vi "Lab_2_START_Arrays_String_ShiftRegisters (3) (1).vi"() -> ()   [LabVIEW 2025]
panel:
  out "BPM":cluster{"Time":timestamp[], "Bpm":i32[]}(graph)
  out "HEART RATE ZONES 2":T1(graph)
  out "HEART RATE ZONES":string[][](array[string])
  in  "Age":i32
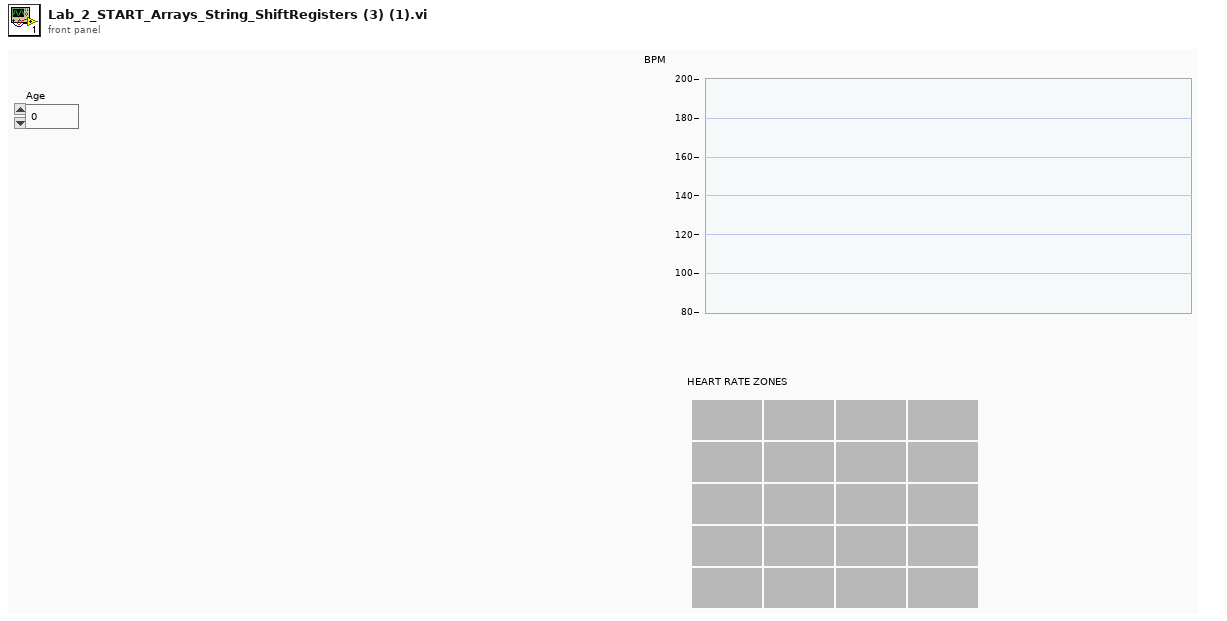
[diagram p1: front panel]
types:
  T1 = cluster{" Total time in Zone (%) ":dbl[], "Heart Rate Zone":i32[]}
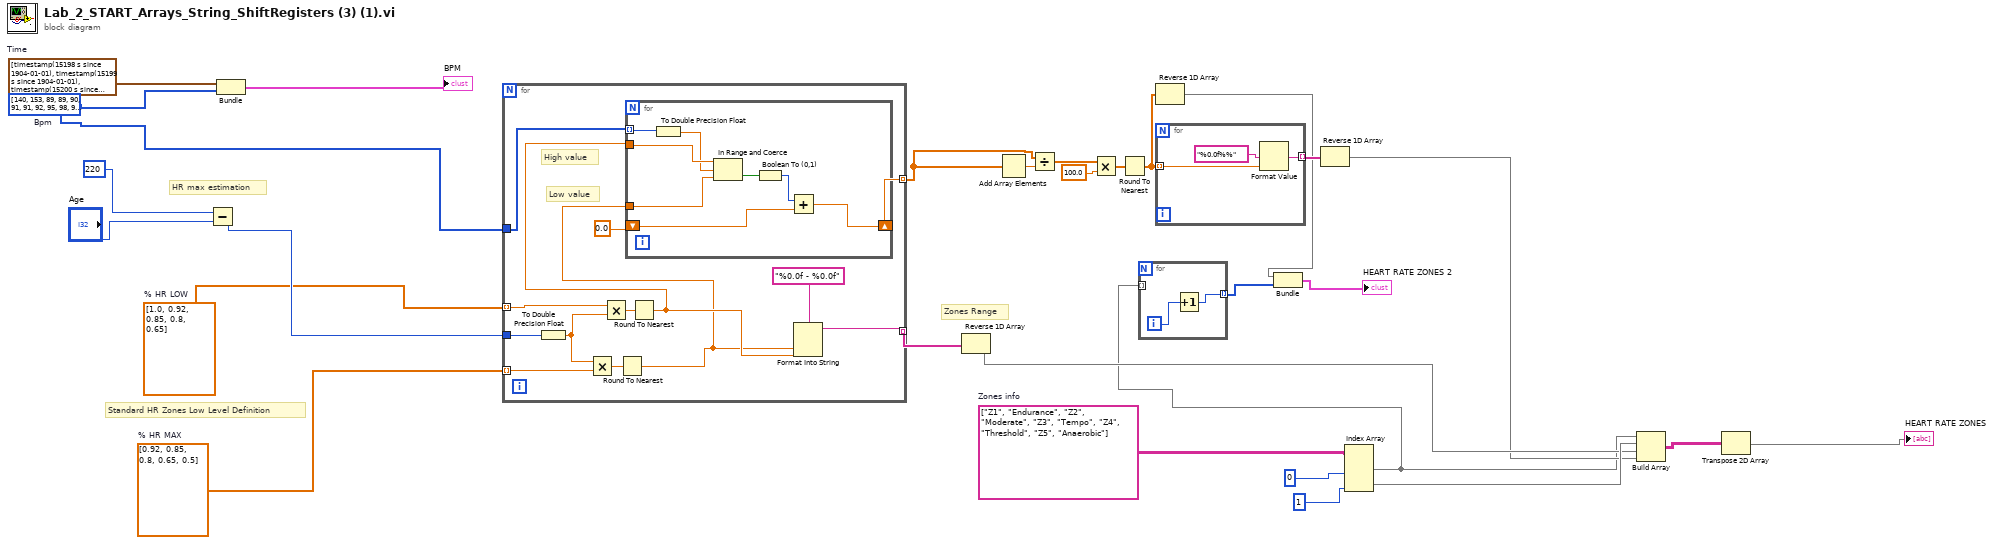
[diagram p0: block diagram]
diagram:
  w24 = dbl[] [1.0, 0.92, 0.85, 0.8, 0.65]  # % HR LOW
  w4 = i32[] [140, 153, 89, 89, 90, 91, 91, 92, 95, 98, 99, 103, 105, 112, 112, 113, 116, 117, 120, 123, 124, 127, 128, 129, 129, 129, 132, 132, 132, 133, 132, 135, 136, 137, 137, 136, 137, 138, 142, 142, 143, 146, 145, 145, 146, 146, 145, 146, 149, 146, 148, 145, 145, 146, 147, 147, 146, 145, 145, 146, 146, 146, 147, 148, 146, 146, 144, 143, 143, 143, 141, 141, 140, 142, 143, 144, 143, 143, 143, 143, 146, 146, 146, 146, 149, 149, 150, 152, 152, 152, 152, 153, 151, 150, 151, 151, 150, 150, 151, 151, 150, 151, 151, 151, 150, 151, 150, 148, 148, 148, 147, 157, 147, 147, 147, 148, 150, 151, 152, 152, 154, 154, 155, 155, 154, 154, 153, 153, 153, 153, 152, 149, 149, 149, 148, 147, 147, 147, 146, 146, 146, 147, 144, 143, 142, 141, 140, 141, 142, 142, 142, 141, 141, 142, 141, 140, 140, 140, 140, 140, 140, 140, 140, 139, 140, 139, 139, 139, 138, 140, 142, 141, 141, 142, 143, 143, 143, 139, 139, 140, 140, 142, 144, 145, 147, 148, 149, 150, 152, 152, 152, 153, 153, 154, 154, 155, 155, 156, 157, 156, 156, 155, 155, 151, 155, 154, 154, 153, 152, 152, 152, 152, 152, 152, 151, 151, 150, 150, 151, 150, 151, 150, 151, 151, 152, 152, 151, 152, 151, 150, 152, 151, 151, 150, 150, 149, 148, 148, 148, 148, 149, 150, 151, 151, 149, 149, 148, 148, 148, 150, 152, 152, 153, 151, 151, 151, 152, 153, 153, 152, 151, 151, 152, 151, 151, 151, 152, 152, 153, 167, 173, 153, 155, 157, 158, 159, 160, 160, 159, 159, 160, 161, 161, 162, 161, 162, 163, 164, 165, 165, 164, 165, 165, 166, 167, 167, 167, 167, 168, 167, 167, 167, 168, 168, 168, 168, 169, 169, 169, 170, 169, 172, 173, 170, 171, 171, 172, 172, 171, 171, 171, 171, 171, 171, 169, 166, 172, 173, 172, 173, 172, 172, 172, 172, 172, 172, 173, 172, 173, 172, 172, 172, 172, 172, 172, 171, 172, 172, 172, 129, 173, 172, 172, 173, 169, 166, 166, 166, 164, 163, 162, 161, 161, 157, 156, 154, 150, 149, 146, 143, 140, 137, 138, 137, 135, 135, 134, 135, 132, 131, 129, 128, 126, 126, 125, 126, 123, 123, 125, 124, 120, 118, 118, 116, 116, 116, 116, 116, 116, 115, 116, 114, 115, 117, 116, 116, 115, 114, 116, 116, 113, 112, 112, 112, 113, 116, 118, 121, 164, 176, 121, 125, 129, 133, 136, 139, 141, 144, 146, 149, 150, 153, 153, 156, 156, 157, 159, 161, 161, 163, 163, 164, 164, 164, 164, 166, 165, 167, 168, 168, 168, 167, 168, 168, 169, 169, 169, 170, 171, 171, 172, 171, 174, 172, 173, 171, 174, 173, 172, 172, 172, 172, 173, 173, 172, 173, 174, 173, 174, 174, 174, 174, 175, 175, 175, 175, 175, 136, 175, 175, 175, 174, 173, 173, 170, 169, 165, 164, 164, 163, 163, 160, 157, 154, 151, 150, 147, 144, 144, 141, 138, 137, 134, 133, 134, 131, 129, 128, 127, 126, 126, 124, 123, 122, 122, 124, 123, 122, 121, 120, 119, 119, 119, 119, 123, 125, 124, 124, 122, 124, 127, 130, 133, 134, 162, 172, 134, 137, 138, 142, 145, 145, 147, 150, 150, 151, 153, 155, 157, 160, 160, 162, 163, 164, 164, 165, 167, 167, 168, 168, 169, 169, 170, 170, 170, 170, 170, 170, 170, 170, 171, 171, 171, 172, 171, 156, 172, 171, 170, 168, 168, 168, 166, 166, 165, 164, 163, 164, 163, 163, 163, 162, 162, 160, 159, 159, 158, 156, 156, 155, 152, 152, 152, 151, 149, 149, 149, 149, 148, 147, 148, 148, 148, 149, 148, 148, 148, 149, 149, 151, 151, 161, 166, 151, 153, 153, 156, 158, 161, 162, 161, 163, 165, 166, 166, 153, 166, 166, 165, 162, 162, 161, 160, 157, 155, 152, 151, 151, 152, 152, 151, 151, 149, 148, 148, 148, 155, 159, 148, 149, 152, 153, 155, 158, 158, 159, 159, 156, 159, 159, 159, 158, 158, 158, 158, 157, 157, 155, 155, 155, 154, 154, 152, 153, 160, 165, 153, 153, 153, 156, 156, 158, 160, 162, 164, 165, 165, 165, 155, 165, 165, 164, 161, 160, 159, 159, 156, 156, 155, 155, 154, 154, 154, 153, 153, 153, 151, 150, 151, 151, 161, 167, 151, 154, 156, 159, 160, 163, 163, 166, 167, 166, 157, 166, 166, 165, 162, 162, 162, 162, 161, 160, 159, 159, 157, 156, 156, 153, 154, 153, 151, 150, 151, 153, 160, 164, 153, 156, 158, 160, 161, 162, 162, 163, 163, 165, 151, 165, 165, 165, 162, 162, 161, 160, 159, 158, 156, 155, 152, 151, 151, 150, 150, 146, 144, 145, 145, 145, 146, 147, 148, 158, 166, 148, 152, 153, 156, 158, 160, 163, 164, 166, 166, 151, 167, 166, 164, 161, 158, 157, 156, 155, 154, 154, 151, 150, 149, 146, 145, 143, 142, 139, 139, 138, 138, 135, 137, 155, 160, 137, 137, 139, 139, 140, 141, 142, 143, 145, 146, 148, 150, 152, 153, 153, 155, 156, 156, 158, 158, 159, 158, 158, 159, 159, 159, 159, 159, 159, 159, 159, 159, 159, 159, 159, 159, 159, 158, 157, 157, 158, 158, 157, 156, 156, 155, 157, 156, 156, 157, 157, 156, 156, 156, 156, 157, 156, 155, 155, 155, 156, 156, 159, 159, 158, 158, 157, 157, 158, 158, 158, 158, 159, 158, 158, 158, 157, 157, 157, 156, 156, 156, 154, 154, 154, 154, 156, 155, 157, 157, 157, 157, 158, 158, 158, 159]  # Bpm
  w28 = timestamp[] [timestamp(15198 s since 1904-01-01), timestamp(15199 s since 1904-01-01), timestamp(15200 s since 1904-01-01), timestamp(15202 s since 1904-01-01), timestamp(15203 s since 1904-01-01), timestamp(15207 s since 1904-01-01), timestamp(15209 s since 1904-01-01), timestamp(15211 s since 1904-01-01), timestamp(15213 s since 1904-01-01), timestamp(15215 s since 1904-01-01), timestamp(15218 s since 1904-01-01), timestamp(15220 s since 1904-01-01), timestamp(15221 s since 1904-01-01), timestamp(15223 s since 1904-01-01), timestamp(15226 s since 1904-01-01), timestamp(15227 s since 1904-01-01), timestamp(15229 s since 1904-01-01), timestamp(15231 s since 1904-01-01), timestamp(15235 s since 1904-01-01), timestamp(15241 s since 1904-01-01), timestamp(15244 s since 1904-01-01), timestamp(15245 s since 1904-01-01), timestamp(15248 s since 1904-01-01), timestamp(15250 s since 1904-01-01), timestamp(15256 s since 1904-01-01), timestamp(15257 s since 1904-01-01), timestamp(15258 s since 1904-01-01), timestamp(15263 s since 1904-01-01), timestamp(15265 s since 1904-01-01), timestamp(15267 s since 1904-01-01), timestamp(15269 s since 1904-01-01), timestamp(15274 s since 1904-01-01), timestamp(15275 s since 1904-01-01), timestamp(15277 s since 1904-01-01), timestamp(15279 s since 1904-01-01), timestamp(15285 s since 1904-01-01), timestamp(15291 s since 1904-01-01), timestamp(15294 s since 1904-01-01), timestamp(15299 s since 1904-01-01), timestamp(15301 s since 1904-01-01), timestamp(15302 s since 1904-01-01), timestamp(15308 s since 1904-01-01), timestamp(15313 s since 1904-01-01), timestamp(15319 s since 1904-01-01), timestamp(15320 s since 1904-01-01), timestamp(15324 s since 1904-01-01), timestamp(15329 s since 1904-01-01), timestamp(15335 s since 1904-01-01), timestamp(15337 s since 1904-01-01), timestamp(15341 s since 1904-01-01), timestamp(15343 s since 1904-01-01), timestamp(15348 s since 1904-01-01), timestamp(15354 s since 1904-01-01), timestamp(15355 s since 1904-01-01), timestamp(15356 s since 1904-01-01), timestamp(15362 s since 1904-01-01), timestamp(15364 s since 1904-01-01), timestamp(15370 s since 1904-01-01), timestamp(15373 s since 1904-01-01), timestamp(15376 s since 1904-01-01), timestamp(15379 s since 1904-01-01), timestamp(15381 s since 1904-01-01), timestamp(15387 s since 1904-01-01), timestamp(15392 s since 1904-01-01), timestamp(15398 s since 1904-01-01), timestamp(15402 s since 1904-01-01), timestamp(15405 s since 1904-01-01), timestamp(15411 s since 1904-01-01), timestamp(15412 s since 1904-01-01), timestamp(15418 s since 1904-01-01), timestamp(15424 s since 1904-01-01), timestamp(15426 s since 1904-01-01), timestamp(15428 s since 1904-01-01), timestamp(15433 s since 1904-01-01), timestamp(15436 s since 1904-01-01), timestamp(15440 s since 1904-01-01), timestamp(15446 s since 1904-01-01), timestamp(15447 s since 1904-01-01), timestamp(15450 s since 1904-01-01), timestamp(15451 s since 1904-01-01), timestamp(15452 s since 1904-01-01), timestamp(15453 s since 1904-01-01), timestamp(15456 s since 1904-01-01), timestamp(15458 s since 1904-01-01), timestamp(15459 s since 1904-01-01), timestamp(15465 s since 1904-01-01), timestamp(15466 s since 1904-01-01), timestamp(15468 s since 1904-01-01), timestamp(15471 s since 1904-01-01), timestamp(15472 s since 1904-01-01), timestamp(15477 s since 1904-01-01), timestamp(15483 s since 1904-01-01), timestamp(15484 s since 1904-01-01), timestamp(15486 s since 1904-01-01), timestamp(15491 s since 1904-01-01), timestamp(15494 s since 1904-01-01), timestamp(15498 s since 1904-01-01), timestamp(15504 s since 1904-01-01), timestamp(15509 s since 1904-01-01), timestamp(15515 s since 1904-01-01), timestamp(15516 s since 1904-01-01), timestamp(15521 s since 1904-01-01), timestamp(15522 s since 1904-01-01), timestamp(15525 s since 1904-01-01), timestamp(15531 s since 1904-01-01), timestamp(15537 s since 1904-01-01), timestamp(15538 s since 1904-01-01), timestamp(15540 s since 1904-01-01), timestamp(15546 s since 1904-01-01), timestamp(15547 s since 1904-01-01), timestamp(15548 s since 1904-01-01), timestamp(15552 s since 1904-01-01), timestamp(15556 s since 1904-01-01), timestamp(15559 s since 1904-01-01), timestamp(15562 s since 1904-01-01), timestamp(15568 s since 1904-01-01), timestamp(15573 s since 1904-01-01), timestamp(15574 s since 1904-01-01), timestamp(15580 s since 1904-01-01), timestamp(15581 s since 1904-01-01), timestamp(15583 s since 1904-01-01), timestamp(15586 s since 1904-01-01), timestamp(15592 s since 1904-01-01), timestamp(15596 s since 1904-01-01), timestamp(15597 s since 1904-01-01), timestamp(15603 s since 1904-01-01), timestamp(15608 s since 1904-01-01), timestamp(15612 s since 1904-01-01), timestamp(15613 s since 1904-01-01), timestamp(15619 s since 1904-01-01), timestamp(15621 s since 1904-01-01), timestamp(15623 s since 1904-01-01), timestamp(15627 s since 1904-01-01), timestamp(15629 s since 1904-01-01), timestamp(15633 s since 1904-01-01), timestamp(15634 s since 1904-01-01), timestamp(15639 s since 1904-01-01), timestamp(15641 s since 1904-01-01), timestamp(15646 s since 1904-01-01), timestamp(15650 s since 1904-01-01), timestamp(15653 s since 1904-01-01), timestamp(15656 s since 1904-01-01), timestamp(15660 s since 1904-01-01), timestamp(15664 s since 1904-01-01), timestamp(15668 s since 1904-01-01), timestamp(15669 s since 1904-01-01), timestamp(15671 s since 1904-01-01), timestamp(15675 s since 1904-01-01), timestamp(15676 s since 1904-01-01), timestamp(15678 s since 1904-01-01), timestamp(15683 s since 1904-01-01), timestamp(15689 s since 1904-01-01), timestamp(15690 s since 1904-01-01), timestamp(15694 s since 1904-01-01), timestamp(15695 s since 1904-01-01), timestamp(15699 s since 1904-01-01), timestamp(15700 s since 1904-01-01), timestamp(15701 s since 1904-01-01), timestamp(15704 s since 1904-01-01), timestamp(15707 s since 1904-01-01), timestamp(15711 s since 1904-01-01), timestamp(15713 s since 1904-01-01), timestamp(15714 s since 1904-01-01), timestamp(15718 s since 1904-01-01), timestamp(15724 s since 1904-01-01), timestamp(15730 s since 1904-01-01), timestamp(15734 s since 1904-01-01), timestamp(15736 s since 1904-01-01), timestamp(15742 s since 1904-01-01), timestamp(15746 s since 1904-01-01), timestamp(15752 s since 1904-01-01), timestamp(15754 s since 1904-01-01), timestamp(15759 s since 1904-01-01), timestamp(15764 s since 1904-01-01), timestamp(15769 s since 1904-01-01), timestamp(15770 s since 1904-01-01), timestamp(15775 s since 1904-01-01), timestamp(15779 s since 1904-01-01), timestamp(15781 s since 1904-01-01), timestamp(15784 s since 1904-01-01), timestamp(15789 s since 1904-01-01), timestamp(15791 s since 1904-01-01), timestamp(15794 s since 1904-01-01), timestamp(15800 s since 1904-01-01), timestamp(15805 s since 1904-01-01), timestamp(15806 s since 1904-01-01), timestamp(15809 s since 1904-01-01), timestamp(15813 s since 1904-01-01), timestamp(15814 s since 1904-01-01), timestamp(15820 s since 1904-01-01), timestamp(15826 s since 1904-01-01), timestamp(15827 s since 1904-01-01), timestamp(15828 s since 1904-01-01), timestamp(15834 s since 1904-01-01), timestamp(15839 s since 1904-01-01), timestamp(15841 s since 1904-01-01), timestamp(15847 s since 1904-01-01), timestamp(15848 s since 1904-01-01), timestamp(15853 s since 1904-01-01), timestamp(15858 s since 1904-01-01), timestamp(15860 s since 1904-01-01), timestamp(15865 s since 1904-01-01), timestamp(15866 s since 1904-01-01), timestamp(15868 s since 1904-01-01), timestamp(15871 s since 1904-01-01), timestamp(15875 s since 1904-01-01), timestamp(15876 s since 1904-01-01), timestamp(15882 s since 1904-01-01), timestamp(15883 s since 1904-01-01), timestamp(15884 s since 1904-01-01), timestamp(15890 s since 1904-01-01), timestamp(15896 s since 1904-01-01), timestamp(15898 s since 1904-01-01), timestamp(15904 s since 1904-01-01), timestamp(15906 s since 1904-01-01), timestamp(15912 s since 1904-01-01), timestamp(15915 s since 1904-01-01), timestamp(15917 s since 1904-01-01), timestamp(15923 s since 1904-01-01), timestamp(15929 s since 1904-01-01), timestamp(15930 s since 1904-01-01), timestamp(15935 s since 1904-01-01), timestamp(15937 s since 1904-01-01), timestamp(15939 s since 1904-01-01), timestamp(15945 s since 1904-01-01), timestamp(15946 s since 1904-01-01), timestamp(15952 s since 1904-01-01), timestamp(15953 s since 1904-01-01), timestamp(15959 s since 1904-01-01), timestamp(15962 s since 1904-01-01), timestamp(15966 s since 1904-01-01), timestamp(15972 s since 1904-01-01), timestamp(15978 s since 1904-01-01), timestamp(15980 s since 1904-01-01), timestamp(15986 s since 1904-01-01), timestamp(15988 s since 1904-01-01), timestamp(15994 s since 1904-01-01), timestamp(15996 s since 1904-01-01), timestamp(15999 s since 1904-01-01), timestamp(16003 s since 1904-01-01), timestamp(16006 s since 1904-01-01), timestamp(16010 s since 1904-01-01), timestamp(16016 s since 1904-01-01), timestamp(16018 s since 1904-01-01), timestamp(16024 s since 1904-01-01), timestamp(16026 s since 1904-01-01), timestamp(16032 s since 1904-01-01), timestamp(16036 s since 1904-01-01), timestamp(16042 s since 1904-01-01), timestamp(16043 s since 1904-01-01), timestamp(16048 s since 1904-01-01), timestamp(16054 s since 1904-01-01), timestamp(16057 s since 1904-01-01), timestamp(16063 s since 1904-01-01), timestamp(16064 s since 1904-01-01), timestamp(16070 s since 1904-01-01), timestamp(16074 s since 1904-01-01), timestamp(16080 s since 1904-01-01), timestamp(16081 s since 1904-01-01), timestamp(16087 s since 1904-01-01), timestamp(16093 s since 1904-01-01), timestamp(16095 s since 1904-01-01), timestamp(16099 s since 1904-01-01), timestamp(16102 s since 1904-01-01), timestamp(16107 s since 1904-01-01), timestamp(16113 s since 1904-01-01), timestamp(16117 s since 1904-01-01), timestamp(16121 s since 1904-01-01), timestamp(16125 s since 1904-01-01), timestamp(16127 s since 1904-01-01), timestamp(16132 s since 1904-01-01), timestamp(16133 s since 1904-01-01), timestamp(16138 s since 1904-01-01), timestamp(16140 s since 1904-01-01), timestamp(16143 s since 1904-01-01), timestamp(16148 s since 1904-01-01), timestamp(16153 s since 1904-01-01), timestamp(16158 s since 1904-01-01), timestamp(16161 s since 1904-01-01), timestamp(16167 s since 1904-01-01), timestamp(16169 s since 1904-01-01), timestamp(16174 s since 1904-01-01), timestamp(16178 s since 1904-01-01), timestamp(16183 s since 1904-01-01), timestamp(16187 s since 1904-01-01), timestamp(16192 s since 1904-01-01), timestamp(16195 s since 1904-01-01), timestamp(16200 s since 1904-01-01), timestamp(16202 s since 1904-01-01), timestamp(16203 s since 1904-01-01), timestamp(16209 s since 1904-01-01), timestamp(16212 s since 1904-01-01), timestamp(16214 s since 1904-01-01), timestamp(16219 s since 1904-01-01), timestamp(16223 s since 1904-01-01), timestamp(16225 s since 1904-01-01), timestamp(16230 s since 1904-01-01), timestamp(16236 s since 1904-01-01), timestamp(16242 s since 1904-01-01), timestamp(16244 s since 1904-01-01), timestamp(16245 s since 1904-01-01), timestamp(16250 s since 1904-01-01), timestamp(16254 s since 1904-01-01), timestamp(16260 s since 1904-01-01), timestamp(16262 s since 1904-01-01), timestamp(16267 s since 1904-01-01), timestamp(16270 s since 1904-01-01), timestamp(16275 s since 1904-01-01), timestamp(16279 s since 1904-01-01), timestamp(16285 s since 1904-01-01), timestamp(16287 s since 1904-01-01), timestamp(16293 s since 1904-01-01), timestamp(16295 s since 1904-01-01), timestamp(16301 s since 1904-01-01), timestamp(16303 s since 1904-01-01), timestamp(16308 s since 1904-01-01), timestamp(16314 s since 1904-01-01), timestamp(16316 s since 1904-01-01), timestamp(16317 s since 1904-01-01), timestamp(16323 s since 1904-01-01), timestamp(16324 s since 1904-01-01), timestamp(16326 s since 1904-01-01), timestamp(16332 s since 1904-01-01), timestamp(16338 s since 1904-01-01), timestamp(16340 s since 1904-01-01), timestamp(16346 s since 1904-01-01), timestamp(16348 s since 1904-01-01), timestamp(16350 s since 1904-01-01), timestamp(16352 s since 1904-01-01), timestamp(16358 s since 1904-01-01), timestamp(16364 s since 1904-01-01), timestamp(16368 s since 1904-01-01), timestamp(16374 s since 1904-01-01), timestamp(16377 s since 1904-01-01), timestamp(16383 s since 1904-01-01), timestamp(16386 s since 1904-01-01), timestamp(16392 s since 1904-01-01), timestamp(16395 s since 1904-01-01), timestamp(16399 s since 1904-01-01), timestamp(16401 s since 1904-01-01), timestamp(16402 s since 1904-01-01), timestamp(16403 s since 1904-01-01), timestamp(16404 s since 1904-01-01), timestamp(16407 s since 1904-01-01), timestamp(16408 s since 1904-01-01), timestamp(16409 s since 1904-01-01), timestamp(16410 s since 1904-01-01), timestamp(16411 s since 1904-01-01), timestamp(16412 s since 1904-01-01), timestamp(16416 s since 1904-01-01), timestamp(16417 s since 1904-01-01), timestamp(16419 s since 1904-01-01), timestamp(16423 s since 1904-01-01), timestamp(16427 s since 1904-01-01), timestamp(16430 s since 1904-01-01), timestamp(16431 s since 1904-01-01), timestamp(16434 s since 1904-01-01), timestamp(16437 s since 1904-01-01), timestamp(16443 s since 1904-01-01), timestamp(16445 s since 1904-01-01), timestamp(16446 s since 1904-01-01), timestamp(16448 s since 1904-01-01), timestamp(16449 s since 1904-01-01), timestamp(16450 s since 1904-01-01), timestamp(16456 s since 1904-01-01), timestamp(16457 s since 1904-01-01), timestamp(16460 s since 1904-01-01), timestamp(16461 s since 1904-01-01), timestamp(16464 s since 1904-01-01), timestamp(16466 s since 1904-01-01), timestamp(16469 s since 1904-01-01), timestamp(16470 s since 1904-01-01), timestamp(16471 s since 1904-01-01), timestamp(16476 s since 1904-01-01), timestamp(16478 s since 1904-01-01), timestamp(16479 s since 1904-01-01), timestamp(16483 s since 1904-01-01), timestamp(16485 s since 1904-01-01), timestamp(16488 s since 1904-01-01), timestamp(16491 s since 1904-01-01), timestamp(16496 s since 1904-01-01), timestamp(16500 s since 1904-01-01), timestamp(16502 s since 1904-01-01), timestamp(16503 s since 1904-01-01), timestamp(16508 s since 1904-01-01), timestamp(16512 s since 1904-01-01), timestamp(16513 s since 1904-01-01), timestamp(16519 s since 1904-01-01), timestamp(16521 s since 1904-01-01), timestamp(16527 s since 1904-01-01), timestamp(16532 s since 1904-01-01), timestamp(16538 s since 1904-01-01), timestamp(16540 s since 1904-01-01), timestamp(16543 s since 1904-01-01), timestamp(16545 s since 1904-01-01), timestamp(16547 s since 1904-01-01), timestamp(16553 s since 1904-01-01), timestamp(16554 s since 1904-01-01), timestamp(16558 s since 1904-01-01), timestamp(16564 s since 1904-01-01), timestamp(16566 s since 1904-01-01), timestamp(16568 s since 1904-01-01), timestamp(16571 s since 1904-01-01), timestamp(16574 s since 1904-01-01), timestamp(16576 s since 1904-01-01), timestamp(16579 s since 1904-01-01), timestamp(16579 s since 1904-01-01), timestamp(16581 s since 1904-01-01), timestamp(16583 s since 1904-01-01), timestamp(16586 s since 1904-01-01), timestamp(16590 s since 1904-01-01), timestamp(16593 s since 1904-01-01), timestamp(16596 s since 1904-01-01), timestamp(16599 s since 1904-01-01), timestamp(16602 s since 1904-01-01), timestamp(16608 s since 1904-01-01), timestamp(16612 s since 1904-01-01), timestamp(16617 s since 1904-01-01), timestamp(16619 s since 1904-01-01), timestamp(16625 s since 1904-01-01), timestamp(16626 s since 1904-01-01), timestamp(16629 s since 1904-01-01), timestamp(16634 s since 1904-01-01), timestamp(16640 s since 1904-01-01), timestamp(16642 s since 1904-01-01), timestamp(16648 s since 1904-01-01), timestamp(16652 s since 1904-01-01), timestamp(16658 s since 1904-01-01), timestamp(16659 s since 1904-01-01), timestamp(16664 s since 1904-01-01), timestamp(16666 s since 1904-01-01), timestamp(16672 s since 1904-01-01), timestamp(16675 s since 1904-01-01), timestamp(16681 s since 1904-01-01), timestamp(16686 s since 1904-01-01), timestamp(16692 s since 1904-01-01), timestamp(16696 s since 1904-01-01), timestamp(16702 s since 1904-01-01), timestamp(16708 s since 1904-01-01), timestamp(16710 s since 1904-01-01), timestamp(16716 s since 1904-01-01), timestamp(16718 s since 1904-01-01), timestamp(16724 s since 1904-01-01), timestamp(16726 s since 1904-01-01), timestamp(16731 s since 1904-01-01), timestamp(16733 s since 1904-01-01), timestamp(16739 s since 1904-01-01), timestamp(16743 s since 1904-01-01), timestamp(16746 s since 1904-01-01), timestamp(16750 s since 1904-01-01), timestamp(16755 s since 1904-01-01), timestamp(16761 s since 1904-01-01), timestamp(16766 s since 1904-01-01), timestamp(16767 s since 1904-01-01), timestamp(16769 s since 1904-01-01), timestamp(16770 s since 1904-01-01), timestamp(16773 s since 1904-01-01), timestamp(16774 s since 1904-01-01), timestamp(16779 s since 1904-01-01), timestamp(16780 s since 1904-01-01), timestamp(16785 s since 1904-01-01), timestamp(16786 s since 1904-01-01), timestamp(16791 s since 1904-01-01), timestamp(16794 s since 1904-01-01), timestamp(16798 s since 1904-01-01), timestamp(16800 s since 1904-01-01), timestamp(16804 s since 1904-01-01), timestamp(16809 s since 1904-01-01), timestamp(16814 s since 1904-01-01), timestamp(16816 s since 1904-01-01), timestamp(16822 s since 1904-01-01), timestamp(16824 s since 1904-01-01), timestamp(16830 s since 1904-01-01), timestamp(16830 s since 1904-01-01), timestamp(16831 s since 1904-01-01), timestamp(16834 s since 1904-01-01), timestamp(16835 s since 1904-01-01), timestamp(16836 s since 1904-01-01), timestamp(16839 s since 1904-01-01), timestamp(16840 s since 1904-01-01), timestamp(16846 s since 1904-01-01), timestamp(16848 s since 1904-01-01), timestamp(16849 s since 1904-01-01), timestamp(16851 s since 1904-01-01), timestamp(16853 s since 1904-01-01), timestamp(16857 s since 1904-01-01), timestamp(16861 s since 1904-01-01), timestamp(16864 s since 1904-01-01), timestamp(16867 s since 1904-01-01), timestamp(16869 s since 1904-01-01), timestamp(16874 s since 1904-01-01), timestamp(16879 s since 1904-01-01), timestamp(16880 s since 1904-01-01), timestamp(16884 s since 1904-01-01), timestamp(16887 s since 1904-01-01), timestamp(16889 s since 1904-01-01), timestamp(16895 s since 1904-01-01), timestamp(16899 s since 1904-01-01), timestamp(16905 s since 1904-01-01), timestamp(16907 s since 1904-01-01), timestamp(16910 s since 1904-01-01), timestamp(16916 s since 1904-01-01), timestamp(16922 s since 1904-01-01), timestamp(16925 s since 1904-01-01), timestamp(16926 s since 1904-01-01), timestamp(16932 s since 1904-01-01), timestamp(16934 s since 1904-01-01), timestamp(16935 s since 1904-01-01), timestamp(16939 s since 1904-01-01), timestamp(16942 s since 1904-01-01), timestamp(16948 s since 1904-01-01), timestamp(16952 s since 1904-01-01), timestamp(16954 s since 1904-01-01), timestamp(16960 s since 1904-01-01), timestamp(16966 s since 1904-01-01), timestamp(16967 s since 1904-01-01), timestamp(16973 s since 1904-01-01), timestamp(16975 s since 1904-01-01), timestamp(16980 s since 1904-01-01), timestamp(16982 s since 1904-01-01), timestamp(16988 s since 1904-01-01), timestamp(16993 s since 1904-01-01), timestamp(16996 s since 1904-01-01), timestamp(16999 s since 1904-01-01), timestamp(17001 s since 1904-01-01), timestamp(17005 s since 1904-01-01), timestamp(17009 s since 1904-01-01), timestamp(17010 s since 1904-01-01), timestamp(17010 s since 1904-01-01), timestamp(17012 s since 1904-01-01), timestamp(17013 s since 1904-01-01), timestamp(17016 s since 1904-01-01), timestamp(17020 s since 1904-01-01), timestamp(17021 s since 1904-01-01), timestamp(17023 s since 1904-01-01), timestamp(17027 s since 1904-01-01), timestamp(17028 s since 1904-01-01), timestamp(17030 s since 1904-01-01), timestamp(17036 s since 1904-01-01), timestamp(17042 s since 1904-01-01), timestamp(17044 s since 1904-01-01), timestamp(17049 s since 1904-01-01), timestamp(17052 s since 1904-01-01), timestamp(17058 s since 1904-01-01), timestamp(17064 s since 1904-01-01), timestamp(17070 s since 1904-01-01), timestamp(17071 s since 1904-01-01), timestamp(17077 s since 1904-01-01), timestamp(17083 s since 1904-01-01), timestamp(17088 s since 1904-01-01), timestamp(17094 s since 1904-01-01), timestamp(17100 s since 1904-01-01), timestamp(17106 s since 1904-01-01), timestamp(17112 s since 1904-01-01), timestamp(17114 s since 1904-01-01), timestamp(17119 s since 1904-01-01), timestamp(17120 s since 1904-01-01), timestamp(17126 s since 1904-01-01), timestamp(17128 s since 1904-01-01), timestamp(17134 s since 1904-01-01), timestamp(17136 s since 1904-01-01), timestamp(17137 s since 1904-01-01), timestamp(17143 s since 1904-01-01), timestamp(17144 s since 1904-01-01), timestamp(17147 s since 1904-01-01), timestamp(17151 s since 1904-01-01), timestamp(17153 s since 1904-01-01), timestamp(17153 s since 1904-01-01), timestamp(17158 s since 1904-01-01), timestamp(17162 s since 1904-01-01), timestamp(17163 s since 1904-01-01), timestamp(17165 s since 1904-01-01), timestamp(17169 s since 1904-01-01), timestamp(17175 s since 1904-01-01), timestamp(17176 s since 1904-01-01), timestamp(17182 s since 1904-01-01), timestamp(17185 s since 1904-01-01), timestamp(17191 s since 1904-01-01), timestamp(17193 s since 1904-01-01), timestamp(17199 s since 1904-01-01), timestamp(17201 s since 1904-01-01), timestamp(17203 s since 1904-01-01), timestamp(17209 s since 1904-01-01), timestamp(17215 s since 1904-01-01), timestamp(17218 s since 1904-01-01), timestamp(17224 s since 1904-01-01), timestamp(17226 s since 1904-01-01), timestamp(17232 s since 1904-01-01), timestamp(17237 s since 1904-01-01), timestamp(17243 s since 1904-01-01), timestamp(17249 s since 1904-01-01), timestamp(17253 s since 1904-01-01), timestamp(17259 s since 1904-01-01), timestamp(17262 s since 1904-01-01), timestamp(17268 s since 1904-01-01), timestamp(17269 s since 1904-01-01), timestamp(17272 s since 1904-01-01), timestamp(17278 s since 1904-01-01), timestamp(17283 s since 1904-01-01), timestamp(17289 s since 1904-01-01), timestamp(17291 s since 1904-01-01), timestamp(17297 s since 1904-01-01), timestamp(17299 s since 1904-01-01), timestamp(17305 s since 1904-01-01), timestamp(17306 s since 1904-01-01), timestamp(17312 s since 1904-01-01), timestamp(17315 s since 1904-01-01), timestamp(17321 s since 1904-01-01), timestamp(17326 s since 1904-01-01), timestamp(17332 s since 1904-01-01), timestamp(17333 s since 1904-01-01), timestamp(17333 s since 1904-01-01), timestamp(17334 s since 1904-01-01), timestamp(17335 s since 1904-01-01), timestamp(17338 s since 1904-01-01), timestamp(17340 s since 1904-01-01), timestamp(17343 s since 1904-01-01), timestamp(17346 s since 1904-01-01), timestamp(17347 s since 1904-01-01), timestamp(17352 s since 1904-01-01), timestamp(17356 s since 1904-01-01), timestamp(17361 s since 1904-01-01), timestamp(17363 s since 1904-01-01), timestamp(17363 s since 1904-01-01), timestamp(17364 s since 1904-01-01), timestamp(17368 s since 1904-01-01), timestamp(17369 s since 1904-01-01), timestamp(17370 s since 1904-01-01), timestamp(17371 s since 1904-01-01), timestamp(17374 s since 1904-01-01), timestamp(17377 s since 1904-01-01), timestamp(17383 s since 1904-01-01), timestamp(17386 s since 1904-01-01), timestamp(17387 s since 1904-01-01), timestamp(17389 s since 1904-01-01), timestamp(17393 s since 1904-01-01), timestamp(17399 s since 1904-01-01), timestamp(17402 s since 1904-01-01), timestamp(17408 s since 1904-01-01), timestamp(17411 s since 1904-01-01), timestamp(17417 s since 1904-01-01), timestamp(17423 s since 1904-01-01), timestamp(17423 s since 1904-01-01), timestamp(17424 s since 1904-01-01), timestamp(17429 s since 1904-01-01), timestamp(17431 s since 1904-01-01), timestamp(17437 s since 1904-01-01), timestamp(17443 s since 1904-01-01), timestamp(17444 s since 1904-01-01), timestamp(17450 s since 1904-01-01), timestamp(17453 s since 1904-01-01), timestamp(17453 s since 1904-01-01), timestamp(17456 s since 1904-01-01), timestamp(17462 s since 1904-01-01), timestamp(17464 s since 1904-01-01), timestamp(17470 s since 1904-01-01), timestamp(17472 s since 1904-01-01), timestamp(17478 s since 1904-01-01), timestamp(17480 s since 1904-01-01), timestamp(17486 s since 1904-01-01), timestamp(17492 s since 1904-01-01), timestamp(17498 s since 1904-01-01), timestamp(17501 s since 1904-01-01), timestamp(17502 s since 1904-01-01), timestamp(17508 s since 1904-01-01), timestamp(17513 s since 1904-01-01), timestamp(17513 s since 1904-01-01), timestamp(17514 s since 1904-01-01), timestamp(17515 s since 1904-01-01), timestamp(17519 s since 1904-01-01), timestamp(17520 s since 1904-01-01), timestamp(17525 s since 1904-01-01), timestamp(17526 s since 1904-01-01), timestamp(17531 s since 1904-01-01), timestamp(17533 s since 1904-01-01), timestamp(17538 s since 1904-01-01), timestamp(17542 s since 1904-01-01), timestamp(17543 s since 1904-01-01), timestamp(17543 s since 1904-01-01), timestamp(17547 s since 1904-01-01), timestamp(17552 s since 1904-01-01), timestamp(17553 s since 1904-01-01), timestamp(17555 s since 1904-01-01), timestamp(17556 s since 1904-01-01), timestamp(17559 s since 1904-01-01), timestamp(17560 s since 1904-01-01), timestamp(17561 s since 1904-01-01), timestamp(17566 s since 1904-01-01), timestamp(17567 s since 1904-01-01), timestamp(17571 s since 1904-01-01), timestamp(17577 s since 1904-01-01), timestamp(17580 s since 1904-01-01), timestamp(17586 s since 1904-01-01), timestamp(17587 s since 1904-01-01), timestamp(17593 s since 1904-01-01), timestamp(17596 s since 1904-01-01), timestamp(17602 s since 1904-01-01), timestamp(17603 s since 1904-01-01), timestamp(17603 s since 1904-01-01), timestamp(17606 s since 1904-01-01), timestamp(17609 s since 1904-01-01), timestamp(17612 s since 1904-01-01), timestamp(17614 s since 1904-01-01), timestamp(17618 s since 1904-01-01), timestamp(17621 s since 1904-01-01), timestamp(17626 s since 1904-01-01), timestamp(17628 s since 1904-01-01), timestamp(17633 s since 1904-01-01), timestamp(17633 s since 1904-01-01), timestamp(17639 s since 1904-01-01), timestamp(17643 s since 1904-01-01), timestamp(17644 s since 1904-01-01), timestamp(17647 s since 1904-01-01), timestamp(17651 s since 1904-01-01), timestamp(17655 s since 1904-01-01), timestamp(17656 s since 1904-01-01), timestamp(17657 s since 1904-01-01), timestamp(17658 s since 1904-01-01), timestamp(17660 s since 1904-01-01), timestamp(17664 s since 1904-01-01), timestamp(17665 s since 1904-01-01), timestamp(17671 s since 1904-01-01), timestamp(17672 s since 1904-01-01), timestamp(17673 s since 1904-01-01), timestamp(17679 s since 1904-01-01), timestamp(17685 s since 1904-01-01), timestamp(17687 s since 1904-01-01), timestamp(17693 s since 1904-01-01), timestamp(17693 s since 1904-01-01), timestamp(17696 s since 1904-01-01), timestamp(17699 s since 1904-01-01), timestamp(17704 s since 1904-01-01), timestamp(17705 s since 1904-01-01), timestamp(17710 s since 1904-01-01), timestamp(17712 s since 1904-01-01), timestamp(17714 s since 1904-01-01), timestamp(17719 s since 1904-01-01), timestamp(17723 s since 1904-01-01), timestamp(17723 s since 1904-01-01), timestamp(17725 s since 1904-01-01), timestamp(17729 s since 1904-01-01), timestamp(17730 s since 1904-01-01), timestamp(17731 s since 1904-01-01), timestamp(17732 s since 1904-01-01), timestamp(17733 s since 1904-01-01), timestamp(17734 s since 1904-01-01), timestamp(17735 s since 1904-01-01), timestamp(17741 s since 1904-01-01), timestamp(17745 s since 1904-01-01), timestamp(17746 s since 1904-01-01), timestamp(17748 s since 1904-01-01), timestamp(17752 s since 1904-01-01), timestamp(17753 s since 1904-01-01), timestamp(17756 s since 1904-01-01), timestamp(17761 s since 1904-01-01), timestamp(17766 s since 1904-01-01), timestamp(17772 s since 1904-01-01), timestamp(17774 s since 1904-01-01), timestamp(17780 s since 1904-01-01), timestamp(17782 s since 1904-01-01), timestamp(17783 s since 1904-01-01), timestamp(17783 s since 1904-01-01), timestamp(17788 s since 1904-01-01), timestamp(17789 s since 1904-01-01), timestamp(17793 s since 1904-01-01), timestamp(17796 s since 1904-01-01), timestamp(17802 s since 1904-01-01), timestamp(17805 s since 1904-01-01), timestamp(17808 s since 1904-01-01), timestamp(17812 s since 1904-01-01), timestamp(17813 s since 1904-01-01), timestamp(17813 s since 1904-01-01), timestamp(17819 s since 1904-01-01), timestamp(17821 s since 1904-01-01), timestamp(17825 s since 1904-01-01), timestamp(17827 s since 1904-01-01), timestamp(17833 s since 1904-01-01), timestamp(17836 s since 1904-01-01), timestamp(17837 s since 1904-01-01), timestamp(17838 s since 1904-01-01), timestamp(17842 s since 1904-01-01), timestamp(17843 s since 1904-01-01), timestamp(17847 s since 1904-01-01), timestamp(17853 s since 1904-01-01), timestamp(17856 s since 1904-01-01), timestamp(17858 s since 1904-01-01), timestamp(17859 s since 1904-01-01), timestamp(17863 s since 1904-01-01), timestamp(17864 s since 1904-01-01), timestamp(17865 s since 1904-01-01), timestamp(17866 s since 1904-01-01), timestamp(17869 s since 1904-01-01), timestamp(17873 s since 1904-01-01), timestamp(17873 s since 1904-01-01), timestamp(17874 s since 1904-01-01), timestamp(17880 s since 1904-01-01), timestamp(17886 s since 1904-01-01), timestamp(17888 s since 1904-01-01), timestamp(17890 s since 1904-01-01), timestamp(17896 s since 1904-01-01), timestamp(17900 s since 1904-01-01), timestamp(17906 s since 1904-01-01), timestamp(17909 s since 1904-01-01), timestamp(17913 s since 1904-01-01), timestamp(17917 s since 1904-01-01), timestamp(17921 s since 1904-01-01), timestamp(17923 s since 1904-01-01), timestamp(17925 s since 1904-01-01), timestamp(17930 s since 1904-01-01), timestamp(17934 s since 1904-01-01), timestamp(17935 s since 1904-01-01), timestamp(17941 s since 1904-01-01), timestamp(17947 s since 1904-01-01), timestamp(17948 s since 1904-01-01), timestamp(17952 s since 1904-01-01), timestamp(17957 s since 1904-01-01), timestamp(17963 s since 1904-01-01), timestamp(17965 s since 1904-01-01), timestamp(17971 s since 1904-01-01), timestamp(17974 s since 1904-01-01), timestamp(17980 s since 1904-01-01), timestamp(17984 s since 1904-01-01), timestamp(17989 s since 1904-01-01), timestamp(17995 s since 1904-01-01), timestamp(17997 s since 1904-01-01), timestamp(18002 s since 1904-01-01), timestamp(18004 s since 1904-01-01), timestamp(18009 s since 1904-01-01), timestamp(18010 s since 1904-01-01), timestamp(18014 s since 1904-01-01), timestamp(18020 s since 1904-01-01), timestamp(18022 s since 1904-01-01), timestamp(18028 s since 1904-01-01), timestamp(18030 s since 1904-01-01), timestamp(18031 s since 1904-01-01), timestamp(18035 s since 1904-01-01), timestamp(18039 s since 1904-01-01), timestamp(18040 s since 1904-01-01), timestamp(18046 s since 1904-01-01), timestamp(18052 s since 1904-01-01), timestamp(18055 s since 1904-01-01), timestamp(18061 s since 1904-01-01), timestamp(18062 s since 1904-01-01), timestamp(18068 s since 1904-01-01), timestamp(18074 s since 1904-01-01), timestamp(18075 s since 1904-01-01), timestamp(18081 s since 1904-01-01), timestamp(18087 s since 1904-01-01), timestamp(18088 s since 1904-01-01), timestamp(18089 s since 1904-01-01), timestamp(18093 s since 1904-01-01), timestamp(18099 s since 1904-01-01), timestamp(18101 s since 1904-01-01), timestamp(18107 s since 1904-01-01), timestamp(18110 s since 1904-01-01), timestamp(18116 s since 1904-01-01), timestamp(18117 s since 1904-01-01), timestamp(18123 s since 1904-01-01), timestamp(18125 s since 1904-01-01), timestamp(18130 s since 1904-01-01), timestamp(18132 s since 1904-01-01), timestamp(18133 s since 1904-01-01), timestamp(18139 s since 1904-01-01), timestamp(18140 s since 1904-01-01), timestamp(18145 s since 1904-01-01), timestamp(18147 s since 1904-01-01), timestamp(18149 s since 1904-01-01), timestamp(18155 s since 1904-01-01), timestamp(18157 s since 1904-01-01), timestamp(18162 s since 1904-01-01), timestamp(18163 s since 1904-01-01), timestamp(18169 s since 1904-01-01), timestamp(18175 s since 1904-01-01), timestamp(18176 s since 1904-01-01), timestamp(18177 s since 1904-01-01), timestamp(18183 s since 1904-01-01), timestamp(18184 s since 1904-01-01), timestamp(18190 s since 1904-01-01), timestamp(18193 s since 1904-01-01), timestamp(18199 s since 1904-01-01), timestamp(18200 s since 1904-01-01), timestamp(18204 s since 1904-01-01), timestamp(18206 s since 1904-01-01), timestamp(18212 s since 1904-01-01), timestamp(18213 s since 1904-01-01), timestamp(18217 s since 1904-01-01), timestamp(18218 s since 1904-01-01), timestamp(18219 s since 1904-01-01), timestamp(18221 s since 1904-01-01)]  # Time
  w17 = string[][] [["Z1", "Endurance"], ["Z2", "Moderate"], ["Z3", "Tempo"], ["Z4", "Threshold"], ["Z5", "Anaerobic"]]  # Zones info
  w23 = dbl[] [0.92, 0.85, 0.8, 0.65, 0.5]  # % HR MAX
  # "Zones Range"
  # "Standard HR Zones Low Level Definition"
  # "HR max estimation"
  n1 = Subtract(x=220, y="Age") -> (x-y=w25:i32)
  n2 = Bundle("Time"=w28, "Bpm"=w4) -> (→"BPM":cluster{"Time":timestamp[], "Bpm":i32[]})  [unwired: 1 in]
  n3 = for {
    tunnel: w25 -> [w41]
    tunnel: w24 -> [w39] mode=indexing
    tunnel: w23 -> [w38] mode=indexing
    tunnel: [w34] -> w22 mode=indexing
    tunnel: w4 -> [w33]
    tunnel: [w29] -> w2 mode=indexing
    # "Low value"
    # "High value"
    n4 = To Double Precision Float(number=w41) -> (double precision float=w40:dbl)
    n5 = Multiply(x=w40, y=w38) -> (x*y=w36:dbl)
    n6 = Multiply(x=w39, y=w40) -> (x*y=w37:dbl)
    n7 = Round To Nearest(number=w36) -> (nearest integer value=w31:dbl)
    n8 = Round To Nearest(number=w37) -> (nearest integer value=w32:dbl)
    n9 = for {
      tunnel: w33 -> [w47] mode=indexing
      tunnel: w32 -> [w49]
      tunnel: w31 -> [w48]
      shift-right: [w44] -> w29
      shift-left: 0.0 -> [w45]
      n10 = To Double Precision Float(number=w47) -> (double precision float=w46:dbl)
      n11 = In Range and Coerce(upper limit=w49, x=w46, lower limit=w48) -> (In Range?=w43:bool)  [unwired: 1 out]
      n12 = Boolean To (0,1)(Boolean=w43) -> (0, 1=w42:i16)
      n13 = Add(x=w42, y=w45) -> (x+y=w44:dbl)
    }
    n14 = Format Into String(format string="%0.0f - %0.0f", w31, w32) -> (resulting string=w34:string)  [unwired: 2 in, 1 out]
  }
  n15 = Reverse 1D Array(array=w22) -> (reversed array=w13:string[])
  n16 = Add Array Elements(numeric array=w2) -> (sum=w1:dbl)
  n17 = Divide(x=w2, y=w1) -> (x/y=w19:dbl[])
  n18 = Multiply(x=w19, y=100.0) -> (x*y=w18:dbl[])
  n19 = Round To Nearest(number=w18) -> (nearest integer value=w6:dbl[])
  n20 = Reverse 1D Array(array=w6) -> (reversed array=w5:dbl[])
  n21 = for {
    tunnel: w6 -> [w52] mode=indexing
    tunnel: [w50] -> w20 mode=indexing
    n22 = Format Value(format string="%0.0f%%", value (0)=w52) -> (output string=w50:string)  [unwired: 1 in]
  }
  n23 = Reverse 1D Array(array=w20) -> (reversed array=w10:string[])
  n24 = Index Array(array=w17, index (col) #1=0 ("index (col)"), index (col) #2=1 ("index (col)")) -> (element #1=w9:string[], element #2=w14:string[])  [unwired: 2 in]
  n25 = for {
    tunnel: w9 -> [_] mode=indexing
    tunnel: [w53] -> w7 mode=indexing
    i -> [w54]
    n26 = Increment(x=w54) -> (x+1=w53:i32)
  }
  n27 = Bundle(w5, w7) -> (→"HEART RATE ZONES 2":cluster{dbl[], i32[]})  [unwired: 1 in]
  n28 = Build Array(w9, w14, w13, w10) -> (w12:string[][])
  n29 = Transpose 2D Array(2D array=w12) -> (transposed array=→"HEART RATE ZONES":string[][])
